vi "Create IO Arrays.vi"(8 "error in":errorcluster, 11 "DIG_IO in":refnum<class "DIG_IO.lvclass">) -> (0 "error out":errorcluster, 3 "DIG_IO out":refnum<class "DIG_IO.lvclass">)   [LabVIEW 2019, in "DIG_IO.lvlib" / "DIG_IO.lvclass"]
uses:
  Library/DIG_IO.lvclass
  Library/DIG_IO.lvclass/DIG_IO.ctl
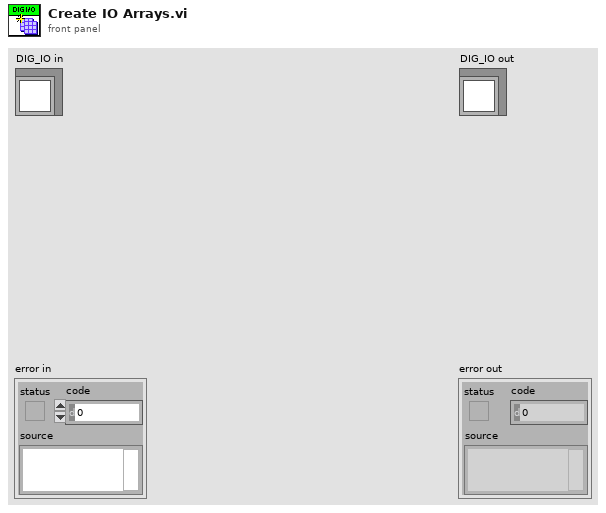
[diagram p1: front panel]
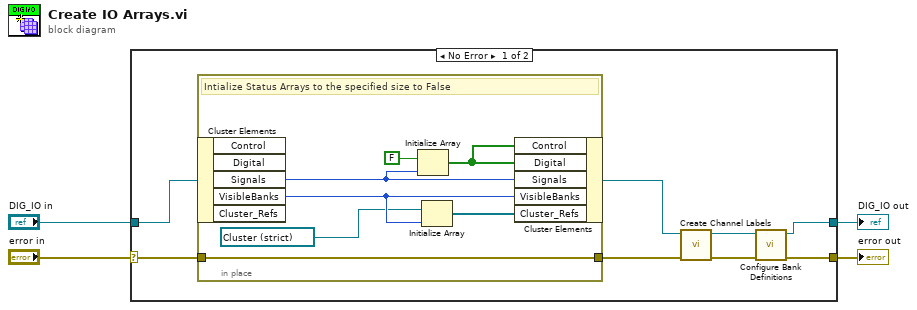
[diagram p0: block diagram]
diagram:
  n1 = case shown="No Error" "error in" {
    selector: "error in" -> [w11 w21]
    tunnel: [w6 w21] -> w3
    tunnel: [w5 w20] -> w1
    tunnel: "DIG_IO in" -> [w12 w20]
    frame No Error {
      n2 = in-place {
        in-place-border: w11 -> [w19]
        in-place-border: [w19] -> w9
        # "Intialize Status Arrays to the specified size to False"
        n3 = in-place-cluster #1(w12) -> ("Signals"=w15:u8, "VisibleBanks"=w18:u8)  [unwired: 3 out]
        n4 = Initialize Array(FALSE, w15) -> (w13:bool[])
        n5 = Initialize Array(refnum<vi> refnum ("Clust_Ref"), w18) -> (w16:refnum<vi>[])
        n6 = in-place-cluster #1("Control"=w13, "Digital"=w13, "Signals"=w15, "VisibleBanks"=w18, "Cluster_Refs"=w16) -> (w10:refnum<class "DIG_IO.lvclass">)
      }
      n7 = call "Create Channel Labels.vi"("error in"=w9, "DIG_IO in"=w10) -> ("error out"=w7:errorcluster, "DIG_IO out"=w8:refnum<class "DIG_IO.lvclass">)  [unwired: 8 in]
      n8 = call "Configure Bank Definitions.vi"("error in (no error)"=w7, "DIG_IO in"=w8) -> ("error out"=w6:errorcluster, "DIG_IO out"=w5:refnum<class "DIG_IO.lvclass">)  [unwired: 8 in]
    }
    frame Error {
    }
  }
  "error out" <- w3
  "DIG_IO out" <- w1
